vi "ABB configure Personel.vi"() -> ()   [LabVIEW 2017]
uses:
  ABB global.vi
panel:
  in  "Edit names":T1
  in  "Enter name":T2
  in  "Personel":i32(listbox)
  in  "Exit":bool
  # "Configure Personel"
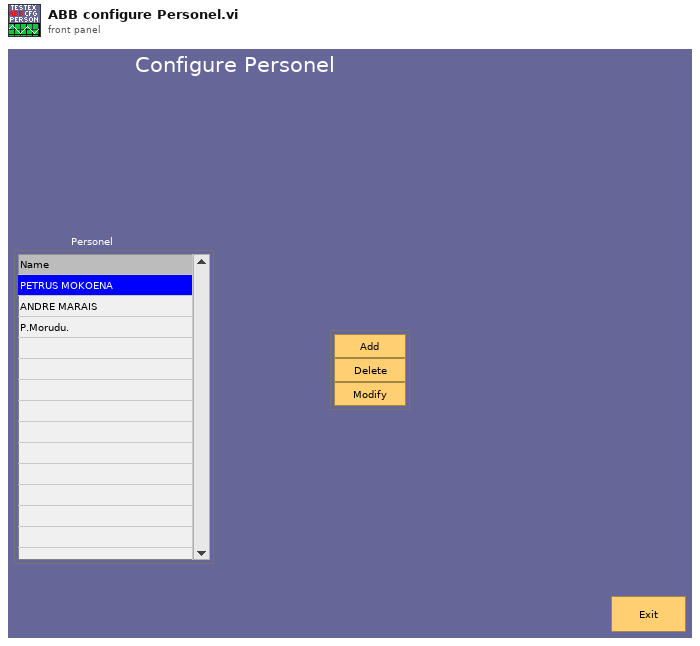
[diagram p1: front panel]
types:
  T1 = cluster{"Add":bool, "Delete":bool, "Modify":bool}
  T2 = cluster{"Name":string, "OK Button":bool, "Cancel Button":bool}
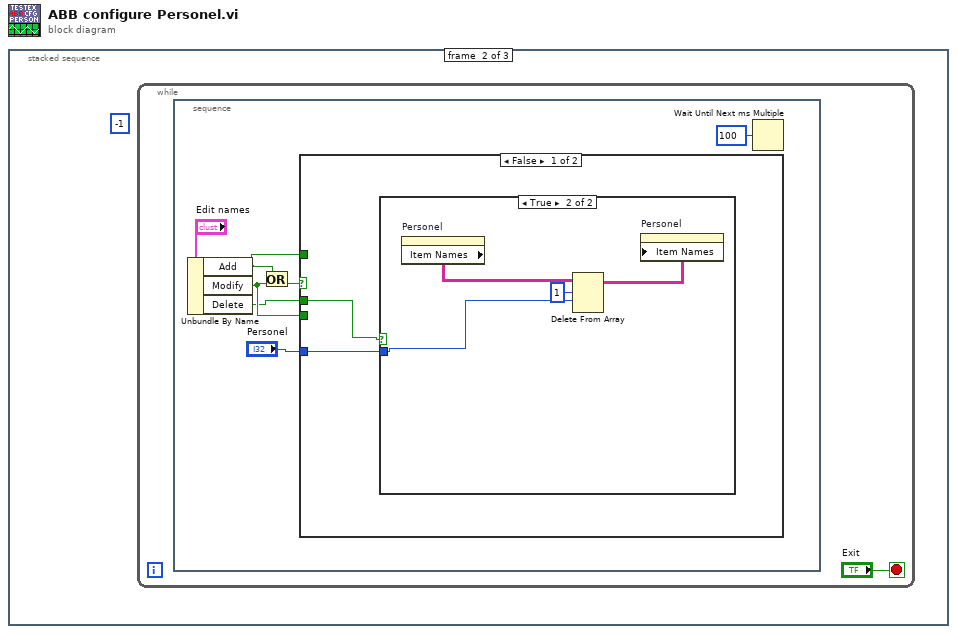
[diagram p0: block diagram]
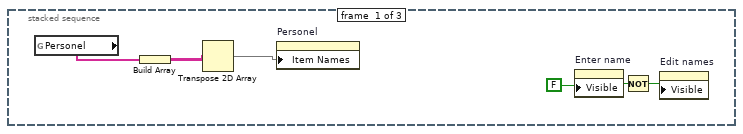
[diagram p2: hidden frame]
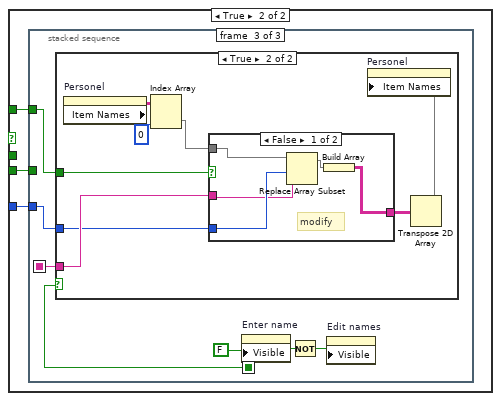
[diagram p4: hidden frame]
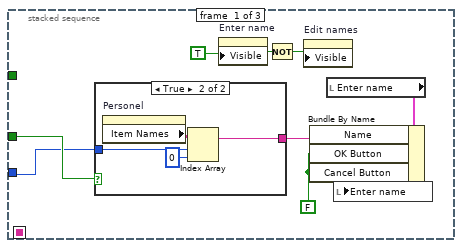
[diagram p5: hidden frame]
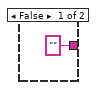
[diagram p6: hidden frame]
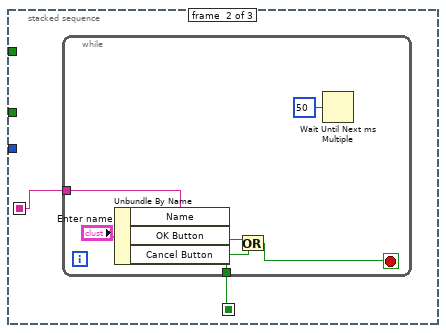
[diagram p7: hidden frame]
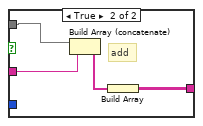
[diagram p9: hidden frame]
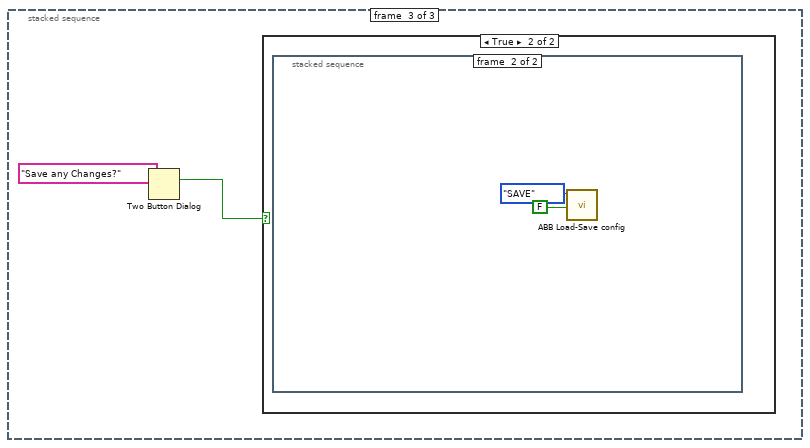
[diagram p10: hidden frame]
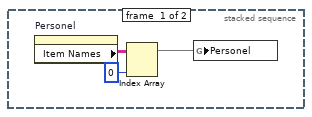
[diagram p12: hidden frame]
diagram:
  n1 = stacked-sequence {
    frame #0 {
      w3 = FALSE ("Visible")
      n2 = global read "ABB global.vi" "Personel"() -> (w5:string[])
      n3 = Build Array(w5) -> (w4:string[][])
      n4 = Transpose 2D Array(2D array=w4) -> (transposed array=w1:string[][])
      n5 = property on="Personel" class="MCListbox (strict)"("Item Names"=w1) -> ()  [unwired: 2 in, 2 out]
      n6 = property on="Enter name" class="Clust (strict)"("Visible"=w3) -> ()  [unwired: 2 in, 2 out]
      n7 = Not(x=w3) -> (.not. x?=w2:bool)
      n8 = property on="Edit names" class="Clust"("Visible"=w2) -> ()  [unwired: 2 in, 2 out]
    }
    frame #1 {
      (unwired) -1 ("Number Values")
      n9 = while {
        stop <- "Exit" stop-if-true
        n10 = stacked-sequence {
          frame #0 {
            n11 = Unbundle By Name("Edit names") -> ("Add"=w10:bool, "Modify"=w8:bool, "Delete"=w7:bool)
            n12 = Or(x=w10, y=w8) -> (x .or. y?=w11:bool)
            n13 = case shown="False" w11 {
              tunnel: w10 -> [_ w22]
              tunnel: "Personel" -> [w14 w21]
              tunnel: w8 -> [_ w20]
              tunnel: w7 -> [w15 _]
              frame False {
                n14 = case shown="True" w15 {
                  tunnel: w14 -> [_ w18]
                  frame False {
                  }
                  frame True {
                    n15 = property on="Personel" class="MCListbox (strict)"() -> ("Item Names"=w19:string[][])  [unwired: 2 in, 2 out]
                    n16 = Delete From Array(array=w19, length=1, index (row)=w18) -> (array with subset deleted=w16:string[][])  [unwired: 1 in, 1 out]
                    n17 = property on="Personel" class="MCListbox (strict)"("Item Names"=w16) -> ()  [unwired: 2 in, 2 out]
                  }
                }
              }
              frame True {
                n18 = stacked-sequence {
                  seq-local: [_ w37 _] -> [_ _ w48]
                  seq-local: [_ w36 _] -> [_ _ w44]
                  tunnel: w22 -> [_ _ w49]
                  tunnel: w21 -> [w27 _ w47]
                  tunnel: w20 -> [w28 _ _]
                  frame #0 {
                    w23 = FALSE
                    w30 = TRUE ("Visible")
                    n19 = case shown="True" w28 {
                      tunnel: w27 -> [_ w33]
                      tunnel: ["" w32] -> w25
                      frame False {
                      }
                      frame True {
                        n20 = property on="Personel" class="MCListbox (strict)"() -> ("Item Names"=w35:string[][])  [unwired: 2 in, 2 out]
                        n21 = Index Array(array=w35, index (row)=w33, index (col)=0 ("disabled index (col)")) -> (element=w32:string)
                      }
                    }
                    n22 = property on="Enter name" class="Clust (strict)"("Visible"=w30) -> ()  [unwired: 2 in, 2 out]
                    n23 = Not(x=w30) -> (.not. x?=w29:bool)
                    n24 = property on="Edit names" class="Clust"("Visible"=w29) -> ()  [unwired: 2 in, 2 out]
                    n25 = local read "Enter name"() -> (w26:T2)
                    n26 = Bundle By Name(cluster=w26, "Name"=w25, "OK Button"=w23, "Cancel Button"=w23) -> (w24:T2)
                    n27 = local write "Enter name"(w24) -> ()
                  }
                  frame #1 {
                    n28 = while {
                      tunnel: [w40] -> w37
                      tunnel: [w38] -> w36
                      stop <- w41 stop-if-true
                      n29 = Unbundle By Name("Enter name") -> ("Name"=w40:string, "OK Button"=w38:bool, "Cancel Button"=w42:bool)
                      n30 = Or(x=w38, y=w42) -> (x .or. y?=w41:bool)
                      n31 = Wait Until Next ms Multiple(millisecond multiple=u32 50) -> ()  [unwired: 1 out]
                    }
                  }
                  frame #2 {
                    w46 = FALSE ("Visible")
                    n32 = case shown="True" w44 {
                      tunnel: w49 -> [_ w55]
                      tunnel: w48 -> [_ w53]
                      tunnel: w47 -> [_ w52]
                      frame False {
                      }
                      frame True {
                        n33 = property on="Personel" class="MCListbox (strict)"() -> ("Item Names"=w57:string[][])  [unwired: 2 in, 2 out]
                        n34 = Index Array(array=w57, index (col)=0 ("disabled index (col)")) -> (element=w54:string[])  [unwired: 1 in]
                        n35 = case shown="False" w55 {
                          tunnel: w54 -> [w62 w66]
                          tunnel: w53 -> [w58 w65]
                          tunnel: [w60 w63] -> w51
                          tunnel: w52 -> [w59 _]
                          frame False {
                            # "modify"
                            n36 = Replace Array Subset(array=w62, new element=w58, index=w59) -> (w61:string[])
                            n37 = Build Array(w61) -> (w60:string[][])
                          }
                          frame True {
                            # "add"
                            n38 = Build Array (concatenate)(w66, w65) -> (w64:string[])
                            n39 = Build Array(w64) -> (w63:string[][])
                          }
                        }
                        n40 = Transpose 2D Array(2D array=w51) -> (transposed array=w50:string[][])
                        n41 = property on="Personel" class="MCListbox (strict)"("Item Names"=w50) -> ()  [unwired: 2 in, 2 out]
                      }
                    }
                    n42 = property on="Enter name" class="Clust (strict)"("Visible"=w46) -> ()  [unwired: 2 in, 2 out]
                    n43 = Not(x=w46) -> (.not. x?=w45:bool)
                    n44 = property on="Edit names" class="Clust"("Visible"=w45) -> ()  [unwired: 2 in, 2 out]
                  }
                }
              }
            }
            n45 = Wait Until Next ms Multiple(millisecond multiple=u32 100) -> ()  [unwired: 1 out]
          }
        }
      }
    }
    frame #2 {
      n46 = Two Button Dialog(message="Save any Changes?") -> (T button?=w68:bool)  [unwired: 2 in]
      n47 = case shown="True" w68 {
        frame False {
        }
        frame True {
          n48 = stacked-sequence {
            frame #0 {
              n49 = property on="Personel" class="MCListbox (strict)"() -> ("Item Names"=w71:string[][])  [unwired: 2 in, 2 out]
              n50 = Index Array(array=w71, index (col)=0 ("disabled index (col)")) -> (element=w69:string[])  [unwired: 1 in]
              n51 = global write "ABB global.vi" "Personel"(w69) -> ()
            }
            frame #1 {
              n52 = call "ABB Load-Save config.vi"("confirm save"=FALSE, "Mode"=enum16{"LOAD", "SAVE"}."SAVE") -> ()  [unwired: 10 in]
            }
          }
        }
      }
    }
  }
